vi "LiftSetLevel.vi"() -> ()   [LabVIEW 2014, in "LiftLib.lvlib"]
uses:
  LiftLib.lvlib
panel:
  in  "index":i32
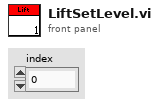
[diagram p1: front panel]
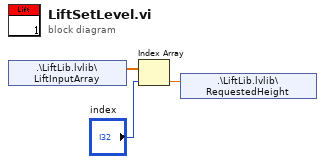
[diagram p0: block diagram]
diagram:
  n1 = shared-variable ".\\LiftLib.lvlib\\LiftInputArray"() -> (w3:dbl[])  [unwired: 1 in, 1 out]
  n2 = Index Array(array=w3, index="index") -> (element=w1:dbl)
  n3 = shared-variable ".\\LiftLib.lvlib\\RequestedHeight"(w1) -> ()  [unwired: 1 in, 1 out]
